vi "clearRead.vi"(3 "ClrCount":u32=10) -> ()   [LabVIEW 2014]
uses:
  ESLSCDLL.dll
panel:
  in  "fftlines":u32=64
  in  "board no":u32=1
  in  "zadr":u32=1
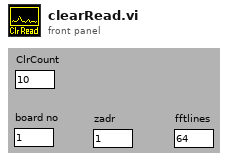
[diagram p1: front panel]
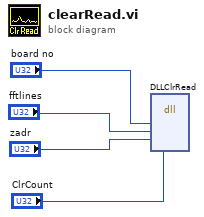
[diagram p0: block diagram]
diagram:
  n1 = dll-call lib="C:/Users/Gerhard/Documents/New64/lv/1cam/board.vis/ESLSCDLL.dll" fn="DLLClrRead"("drvno"="board no", "fftlines"="fftlines", "zadr"="zadr", "CCDClrCount"="ClrCount") -> ()  [unwired: 8 in, 2 out]
